vi "ADO Connection Close.vi"(8 "error in (no error)":errorcluster caption="错误输入（无错误）", 11 "Database Connection 输入":refnum<class "Database Connection.lvclass"> caption="DNL_LabVIEW Object in") -> (0 "error out":errorcluster caption="错误输出")   [LabVIEW 2011, in "Database Connection.lvclass"]
uses:
  Database Connection.lvclass
  Database Connection.lvclass/Database Connection.ctl
panel:
  out "Database Connection 输出":refnum<class "Database Connection.lvclass"> caption="DNL_LabVIEW Object out"
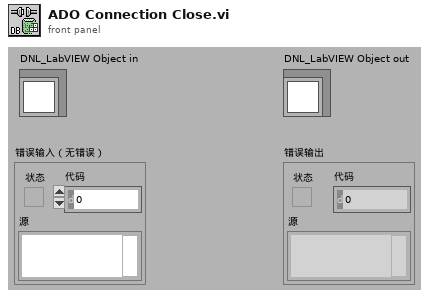
[diagram p1: front panel]
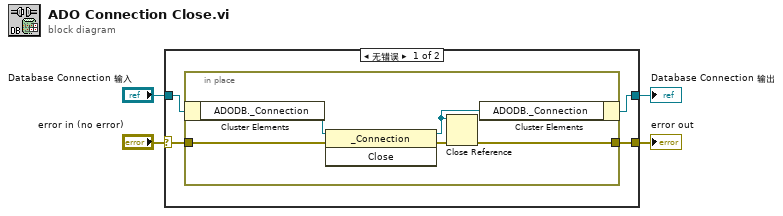
[diagram p0: block diagram]
diagram:
  n1 = case shown="无错误" "error in (no error)" {
    selector: "error in (no error)" -> [w7 w15]
    tunnel: [w6 w15] -> w3
    tunnel: [w5 w14] -> w1
    tunnel: "Database Connection 输入" -> [w8 w14]
    frame No Error {
      n2 = in-place {
        in-place-border: w7 -> [w12]
        in-place-border: [w9] -> w6
        n3 = in-place-cluster #1(w8) -> ("ADODB._Connection"=w13:refnum<k7>)
        n4 = invoke class="_Connection" method="Close"(reference=w13, error in=w12) -> (reference out=w11:refnum<k7>, error out=w10:errorcluster)  [unwired: 1 in, 1 out]
        n5 = Close Reference(reference=w11, error in (no error)=w10) -> (error out=w9:errorcluster)
        n6 = in-place-cluster #1("ADODB._Connection"=w11) -> (w5:refnum<class "Database Connection.lvclass">)
      }
    }
    frame Error {
    }
  }
  "error out" <- w3
  "Database Connection 输出" <- w1
